vi "Set Data Format.vi"(7 "Micropulse # In":i32, 8 "error in (no error)":errorcluster, 9 "Data Formatting":T1 {"Coupling Level" max=4095 step=1}, 11 "Test No.":u32) -> (0 "error out":errorcluster, 3 "Test No. out":u32, 5 "Micropulse # Out":i32)   [LabVIEW 2026, in "MicroPulse_Driver.lvlib"]
uses:
  MicroPulse_Driver.lvlib
  <instrlib>/MicroPulse/Public/Data/Datatypes/MP - data formatting.ctl
  <instrlib>/MicroPulse/Public/Data/Datatypes/MP - amplitude reporting mode.ctl
  <instrlib>/MicroPulse/Public/Data/Datatypes/MP - averaging.ctl
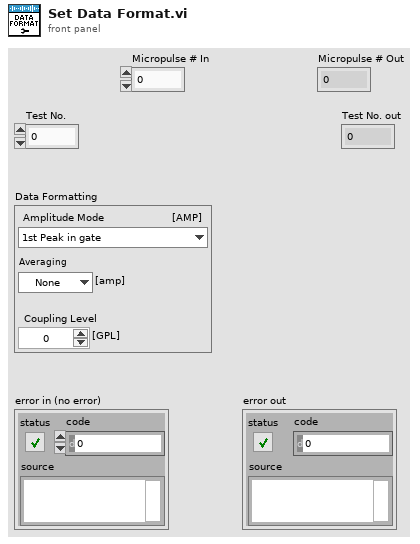
[diagram p1: front panel]
types:
  T1 = typedef "MicroPulse_Driver.lvlib/MP - data formatting.ctl" = cluster{"Amplitude Mode":T2, "Averaging":T3, "Coupling Level":u32}
  T2 = typedef "MicroPulse_Driver.lvlib/MP - amplitude reporting mode.ctl" = enum16{"1st Peak in gate", "Maximum Peak in gate", "All Peaks", "Ascan Data", "1st Threshold Crossing Peak", "Ascan + Peaks", "All Peaks for Multigate", "Peaks + Ascan for Multigate", "Peaks + P_Ascan for Multigate", "Full Matrix Capture"}
  T3 = typedef "MicroPulse_Driver.lvlib/MP - averaging.ctl" = enum16{"None", "2", "4", "8", "16", "32", "64", "128", "256"}
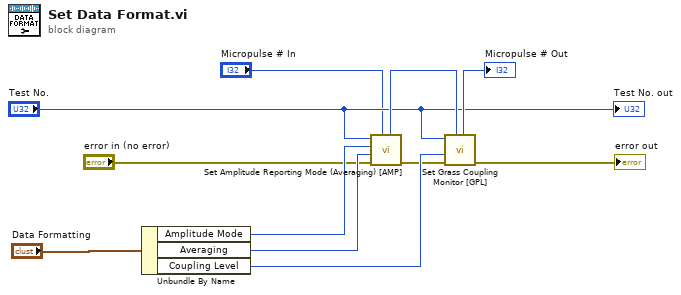
[diagram p0: block diagram]
diagram:
  n1 = Unbundle By Name("Data Formatting") -> ("Amplitude Mode"=w7:T2, "Averaging"=w6:T3, "Coupling Level"=w9:u32)
  n2 = call "Set Amplitude Reporting Mode (Averaging) [AMP].vi"("Micropulse # In"="Micropulse # In", "error in (no error)"="error in (no error)", "Averaging"=w6, "Amplitude Mode"=w7, "Test Number"="Test No.") -> ("error out"=w8:errorcluster, "Micropulse # Out"=w3:i32)  [unwired: 5 in]
  n3 = call "Set Grass Coupling Monitor [GPL].vi"("Micropulse # In"=w3, "error in (no error)"=w8, "Coupling Level"=w9, "Test Number"="Test No.") -> ("error out"=→"error out":errorcluster, "Micropulse # Out"=→"Micropulse # Out":i32)  [unwired: 6 in]
  "Test No. out" <- "Test No."
